vi "TCP_read.vi"(7 "起始地址":u32=10, 8 "error in":errorcluster) -> (0 "error out":errorcluster, 1 "元素":i8)   [LabVIEW 2012]
uses:
  S7Ref.vi
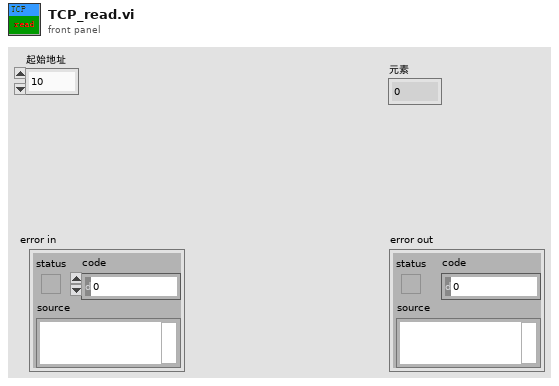
[diagram p1: front panel]
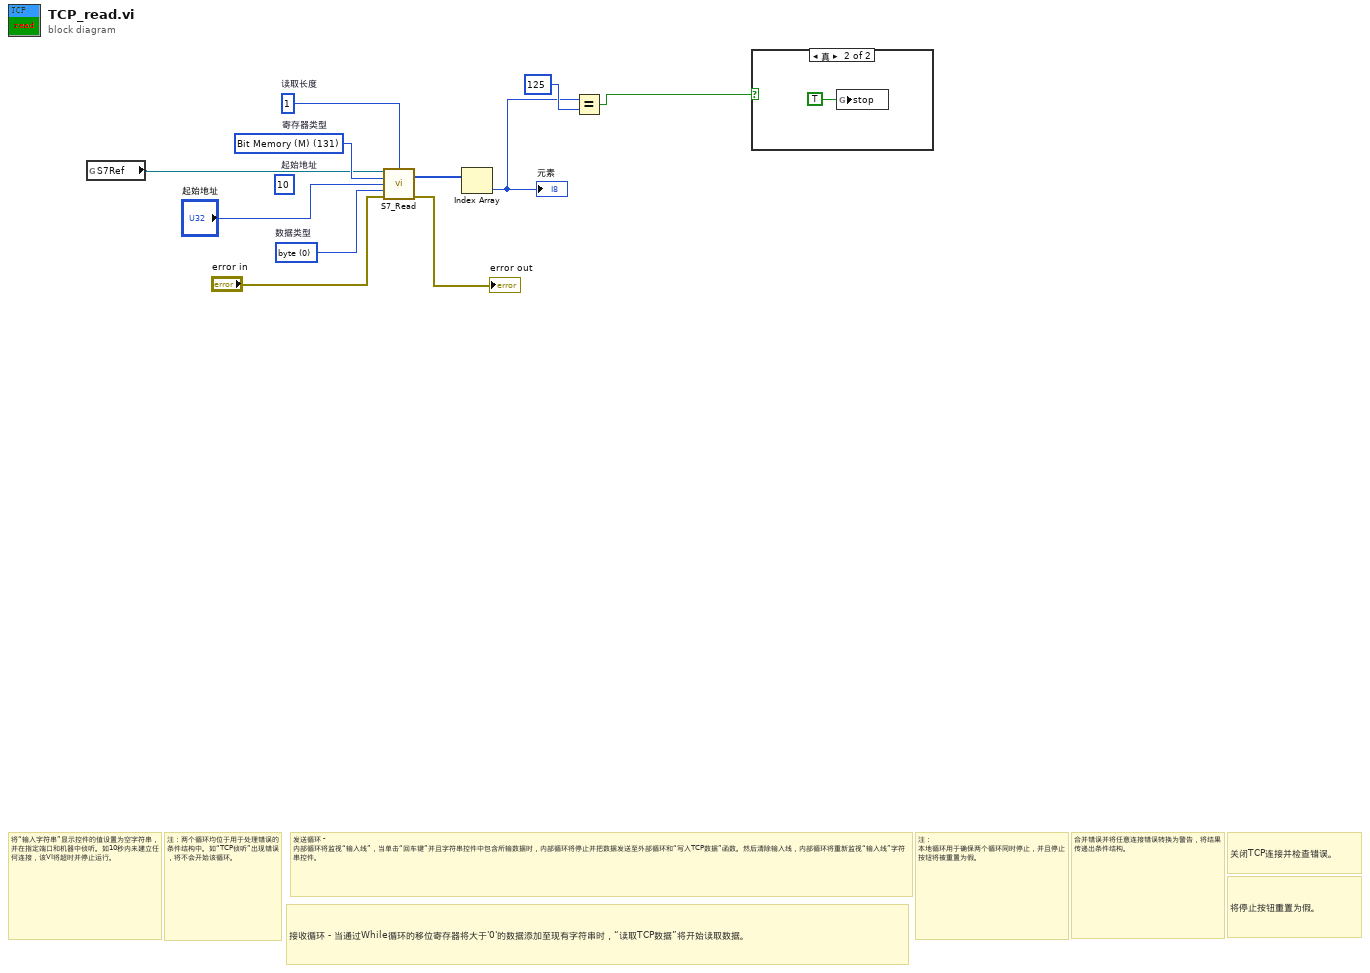
[diagram p0: block diagram]
diagram:
  w10 = u16 0 items=["byte", "word", "Dword"]  # 数据类型
  (unwired) u32 10  # 起始地址
  w11 = u8 131 items=["I/O (P)"=128, "Input (I)"=129, "Output (Q)"=130, "Bit Memory (M)"=131, "Data (DB)"=132, "Instance Data (DI)"=133, "Local Data (L)"=134, "Predecessor Local Data (VL)"=135]  # 寄存器类型
  w9 = u16 1  # 读取长度
  # "将停止按钮重置为假。"
  # "关闭TCP连接并检查错误。"
  # "注：两个循环均位于用于处理错误的条件结构中。如“TCP侦听”出现错误，将不会开始该循环。"
  # "合并错误并将任意连接错误转换为警告，将结果传递出条件结构。"
  # "注： 本地循环用于确保两个循环同时停止，并且停止按钮将被重置为假。"
  # "接收循环 - 当通过While循环的移位寄存器将大于'0'的数据添加至现有字符串时，“读取TCP数据”将开始读取数据。"
  # "发送循环 - 内部循环将监视“输入线”，当单击“回车键”并且字符串控件中包含所输数据时，内部循环将停止并把数据发送至外部循环和“写入TCP数据”函数。然后清除输入线，内部循环将重新监视“输入线”字符串控件。"
  # "将“输入字符串”显示控件的值设置为空字符串，并在指定端口和机器中侦听。如10秒内未建立任何连接，该VI将超时并停止运行。"
  n1 = global read "S7Ref.vi" "S7Ref"() -> (w8:refnum<k5>)
  n2 = call "S7_Read.vi"("TCP"=w8, "读取长度"=w9, "寄存器类型"=w11, "起始地址"="起始地址", "数据类型"=w10, "error in"="error in") -> ("数据"=w7:u32[], "error out"=→"error out":errorcluster)  [unwired: 6 in, 2 out]
  n3 = Index Array(array=w7) -> (element=w4:u32)  [unwired: 1 in]
  "元素" <- w4
  n4 = Equal?(x=w4, y=i8 125) -> (x = y?=w5:bool)
  n5 = case shown="真" w5 {
    frame False {
    }
    frame True {
      n6 = global write "全局 3.vi" "stop"(TRUE ("布尔 1")) -> ()
    }
  }
